vi "6.vi"() -> ()   [LabVIEW 2021]
panel:
  out "difference":u32
  out "square of sums":u32
  out "sum of squares":u32
  in  "n":u32
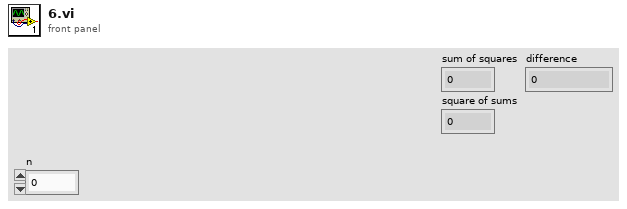
[diagram p1: front panel]
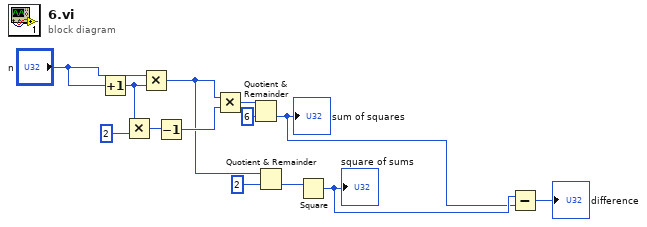
[diagram p0: block diagram]
diagram:
  n1 = Increment(x="n") -> (x+1=w7:u32)
  n2 = Multiply(x=w7, y=u32 2) -> (x*y=w12:u32)
  n3 = Multiply(x="n", y=w7) -> (x*y=w6:u32)
  n4 = Decrement(x=w12) -> (x-1=w11:u32)
  n5 = Multiply(x=w6, y=w11) -> (x*y=w10:u32)
  n6 = Quotient & Remainder(x=w10, y=u32 6) -> (floor(x/y)=w2:u32)  [unwired: 1 out]
  "sum of squares" <- w2
  n7 = Quotient & Remainder(x=w6, y=u32 2) -> (floor(x/y)=w4:u32)  [unwired: 1 out]
  n8 = Square(x=w4) -> (x^2=w3:u32)
  "square of sums" <- w3
  n9 = Subtract(x=w3, y=w2) -> (x-y=→"difference":u32)
